vi "Read All Data.vi"(8 "error in (no error)":errorcluster) -> (0 "error out":errorcluster, 3 "Data Out":refnum<class "Rename.lvclass">)   [LabVIEW 2015, in "Generic Module Library.lvlib" / "Template G_Module.lvlib"]
uses:
  Template G_Module.lvlib
  Data Access Support/Data Actions.ctl
  Module Class/Rename.lvclass
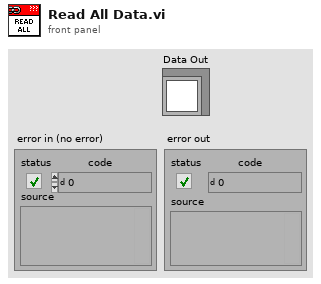
[diagram p1: front panel]
types:
  T1 = typedef "Generic Module Library.lvlib/Template G_Module.lvlib/Data Actions.ctl" = enum16{"Set", "Get"}
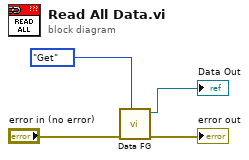
[diagram p0: block diagram]
diagram:
  n1 = call "Data FG.vi"("Data Action"=Data_Actions."Get", "error in (no error)"="error in (no error)") -> ("error out"=→"error out":errorcluster, "Data Out"=→"Data Out":refnum<class "Rename.lvclass">)  [unwired: 8 in]
